vi "State Not a Valid Lua State.vi"(8 "error in (no error)":errorcluster, 11 "Lua in":refnum<class "Lua.lvclass">) -> (0 "error out":errorcluster, 3 "Lua out":refnum<class "Lua.lvclass">)   [LabVIEW 2020, in "Lua for LabVIEW.lvlib" / "Lua.lvclass"]
uses:
  Lua.lvclass
  Lua.lvclass/Lua.ctl
panel:
  out "not a valid state?":bool
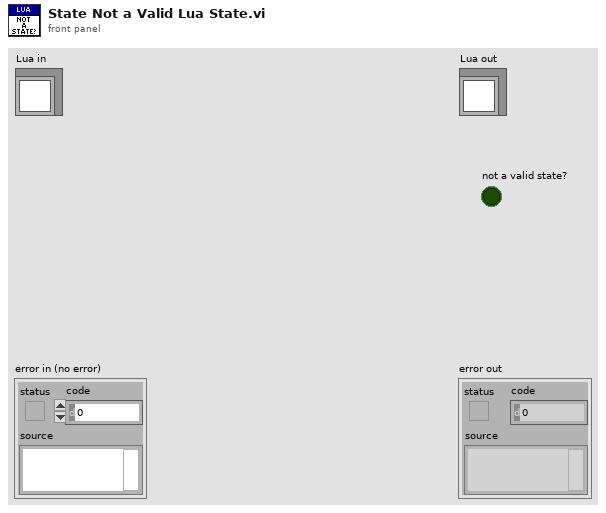
[diagram p1: front panel]
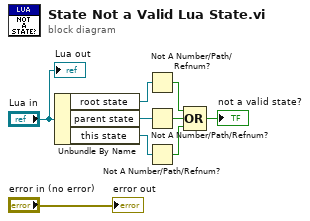
[diagram p0: block diagram]
diagram:
  n1 = Unbundle By Name("Lua in") -> ("root state"=w2:refnum<data-value>, "parent state"=w7:refnum<data-value>, "this state"=w6:refnum<data-value>)
  n2 = Not A Number/Path/Refnum?(number/path/refnum=w2) -> (NaN/Path/Refnum?=w1:bool)
  n3 = Not A Number/Path/Refnum?(number/path/refnum=w7) -> (NaN/Path/Refnum?=w4:bool)
  n4 = Not A Number/Path/Refnum?(number/path/refnum=w6) -> (NaN/Path/Refnum?=w5:bool)
  n5 = Compound Arithmetic op=OR(w1, w4, w5) -> (→"not a valid state?":bool)
  "error out" <- "error in (no error)"
  "Lua out" <- "Lua in"
